vi "test-linear-system-id.vi"(8 "error in (no error)":errorcluster) -> (0 "error out":errorcluster, 3 "All tests passed":bool)   [LabVIEW 2019]
uses:
  <vilib>/Rock Robotics/WPI/ThirdParty/JAS_Junk/TrajLib/LINEAR_SYSTEM.ctl
  <vilib>/Analysis/Matrix/Datatypes/RealMatrix.ctl
  <vilib>/Rock Robotics/WPI/ThirdParty/JAS_Junk/TrajLib/MatBuilder_Create.vi
  <vilib>/Rock Robotics/WPI/ThirdParty/JAS_Junk/TrajLib/LinearSystem_New.vi
  <vilib>/Rock Robotics/WPI/ThirdParty/JAS_Junk/TrajLib/MatrixHelper_Zero.vi
  <vilib>/Rock Robotics/WPI/ThirdParty/JAS_Junk/TrajLib/DCMotor_New.vi
  <vilib>/Rock Robotics/WPI/ThirdParty/JAS_Junk/TrajLib/Units_RotationsPerMinuteToRadiansPerSecond.vi
  <vilib>/Rock Robotics/WPI/ThirdParty/JAS_Junk/TrajLib/MatrixHelper_CoerceSize.vi
  <vilib>/Analysis/7linalg.llb/Create Special Matrix.vi
  <vilib>/Analysis/7linalg.llb/Create Special Real Matrix.vi
  <vilib>/Rock Robotics/WPI/ThirdParty/JAS_Junk/TrajLib/Trajectory_Library.lvlib
  <vilib>/Analysis/Matrix/NI_Matrix.lvlib
panel:
  out "T D 6":bool
  out "T C 6":bool
  out "T B 6":bool
  out "T A 6":bool
  out "DCMotorSystem":T1
  out "T B 5":bool
  out "T A 5":bool
  out "T B 4":bool
  out "T A 4":bool
  out "T D 3":bool
  out "T C 3":bool
  out "T B 3":bool
  out "T A 3":bool
  out "T D 2":bool
  out "T C 2":bool
  out "T B 2":bool
  out "T A 2":bool
  out "T D 1":bool
  out "T C 1":bool
  out "T B 1":bool
  out "T A 1":bool
  out "IdentifyVelocitySystem":T1
  out "IdentifyPositionSystem":T1
  out "FlyWheel":T1
  out "DriveTrain":T1
  out "Elevator":T1
  # "A  = -10.14132, 3.06598, \n            3.06598, -10.14132\n\nB =    4.2590,   -1.28762, \n         -1.2876,   4.2590\n\nC =   1.0,   0.0, \n          0.0,  1.0;\n\nD =   0.0,   0.0, \n          0.0,   0.0"
  # "A   = (0, 1, \n               0, -99.05473)\n\n     B = (0, \n            20.8)\n\n   C   = 1, 0\n\n    D = 0"
  # "A = -26.87032\n\nB = 1354.166667;\n\nC = 1\n\nD = 0"
  # "A =   0, 1, \n         0, -1 / 0.5\n\nB =  0, \n        1 / 0.5"
  # "A =   -1.0 / 0.5\n\nB = 1 / 0.5"
  # "<States,States>"
  # "<States,Inputs>"
  # "<Outputs,States>"
  # "<Outputs,Inputs>"
  # "<States,States>"
  # "<States,Inputs>"
  # "<Outputs,States>"
  # "<Outputs,Inputs>"
  # "<States,States>"
  # "<States,Inputs>"
  # "<Outputs,States>"
  # "<Outputs,Inputs>"
  # "<States,States>"
  # "<States,Inputs>"
  # "<Outputs,States>"
  # "<Outputs,Inputs>"
  # "<States,States>"
  # "<States,Inputs>"
  # "<Outputs,States>"
  # "<Outputs,Inputs>"
  # "<States,States>"
  # "<States,Inputs>"
  # "<Outputs,States>"
  # "<Outputs,Inputs>"
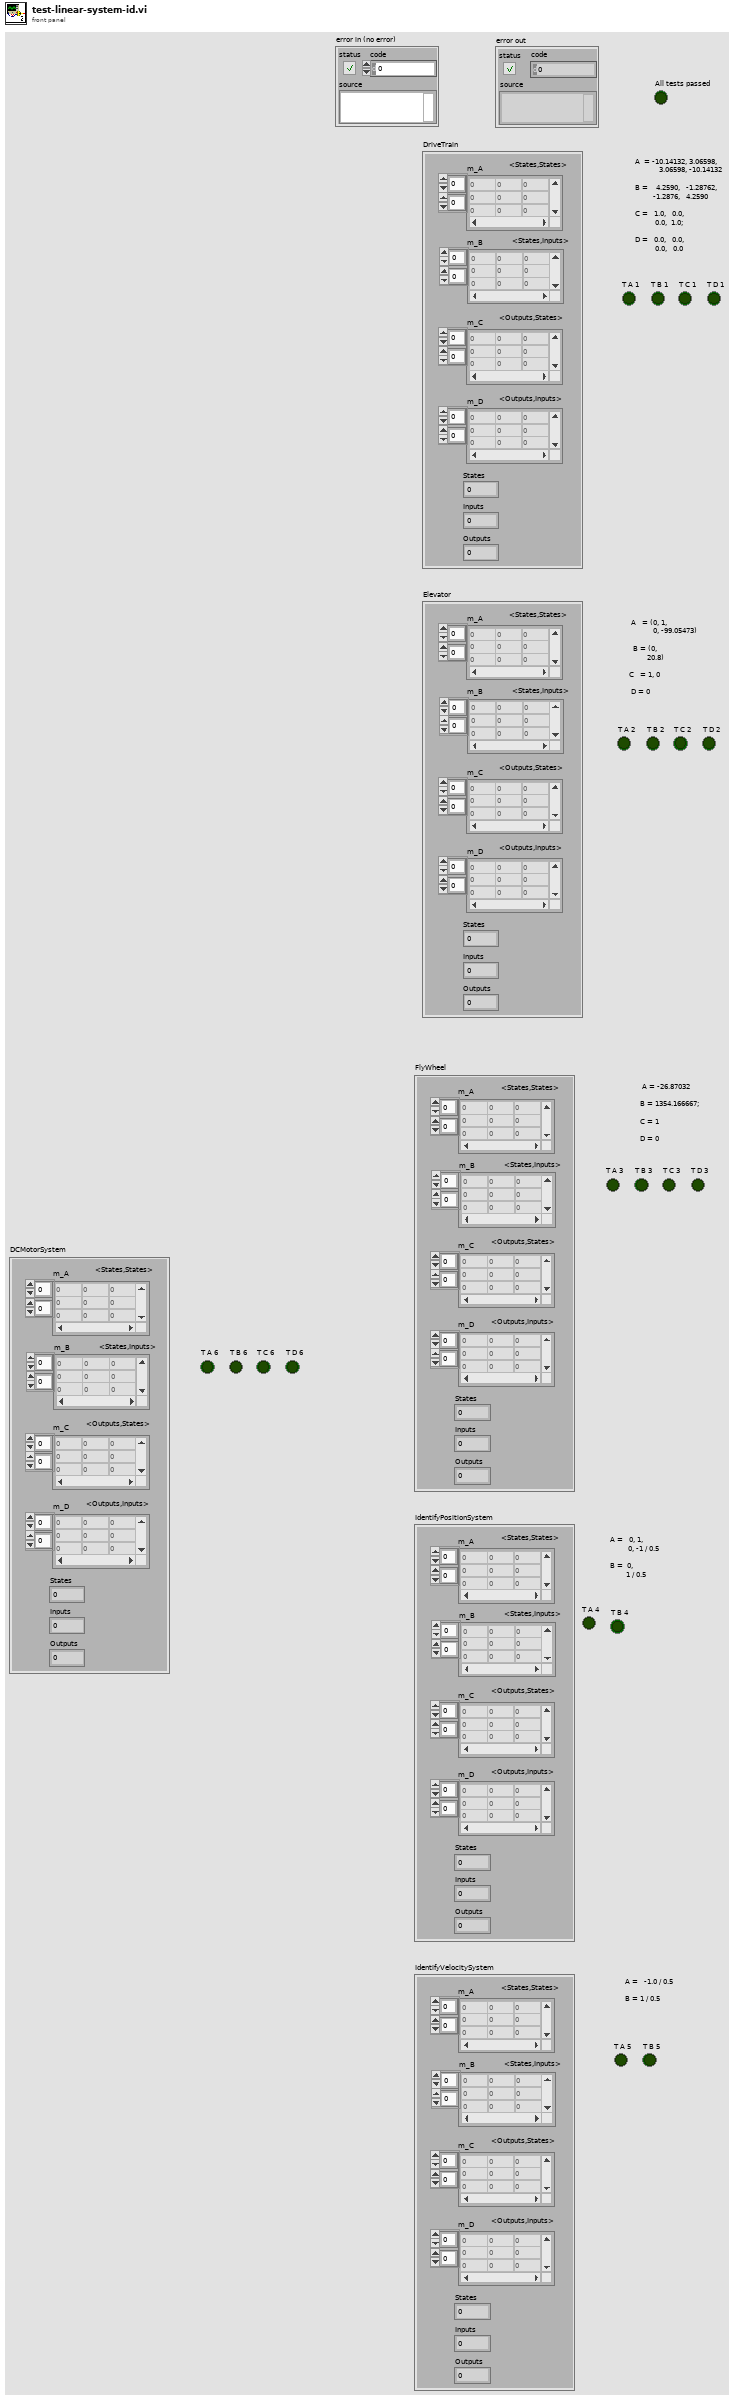
[diagram p1: front panel]
types:
  T1 = typedef "Trajectory_Library.lvlib/LINEAR_SYSTEM.ctl" = cluster{"m_A":T2, "m_B":T2, "m_C":T2, "m_D":T2, "States":i32, "Inputs":i32, "Outputs":i32}
  T2 = typedef "NI_Matrix.lvlib/RealMatrix.ctl" = dbl[][]
  T3 = typedef "Trajectory_Library.lvlib/DCMOTOR.CTL" = cluster{"nominalVoltage_Volts":dbl, "StallTorque_NM":dbl, "StallCurrent_Amps":dbl, "FreeCurrent_Amps":dbl, "FreeSpeed_RadPerSec":dbl, "R_Ohms":dbl, "KvINV_RadPerSecPerVolt":dbl, "Kt_NMPerAmp":dbl, "L_H":dbl, "Jr_KgM2":dbl}
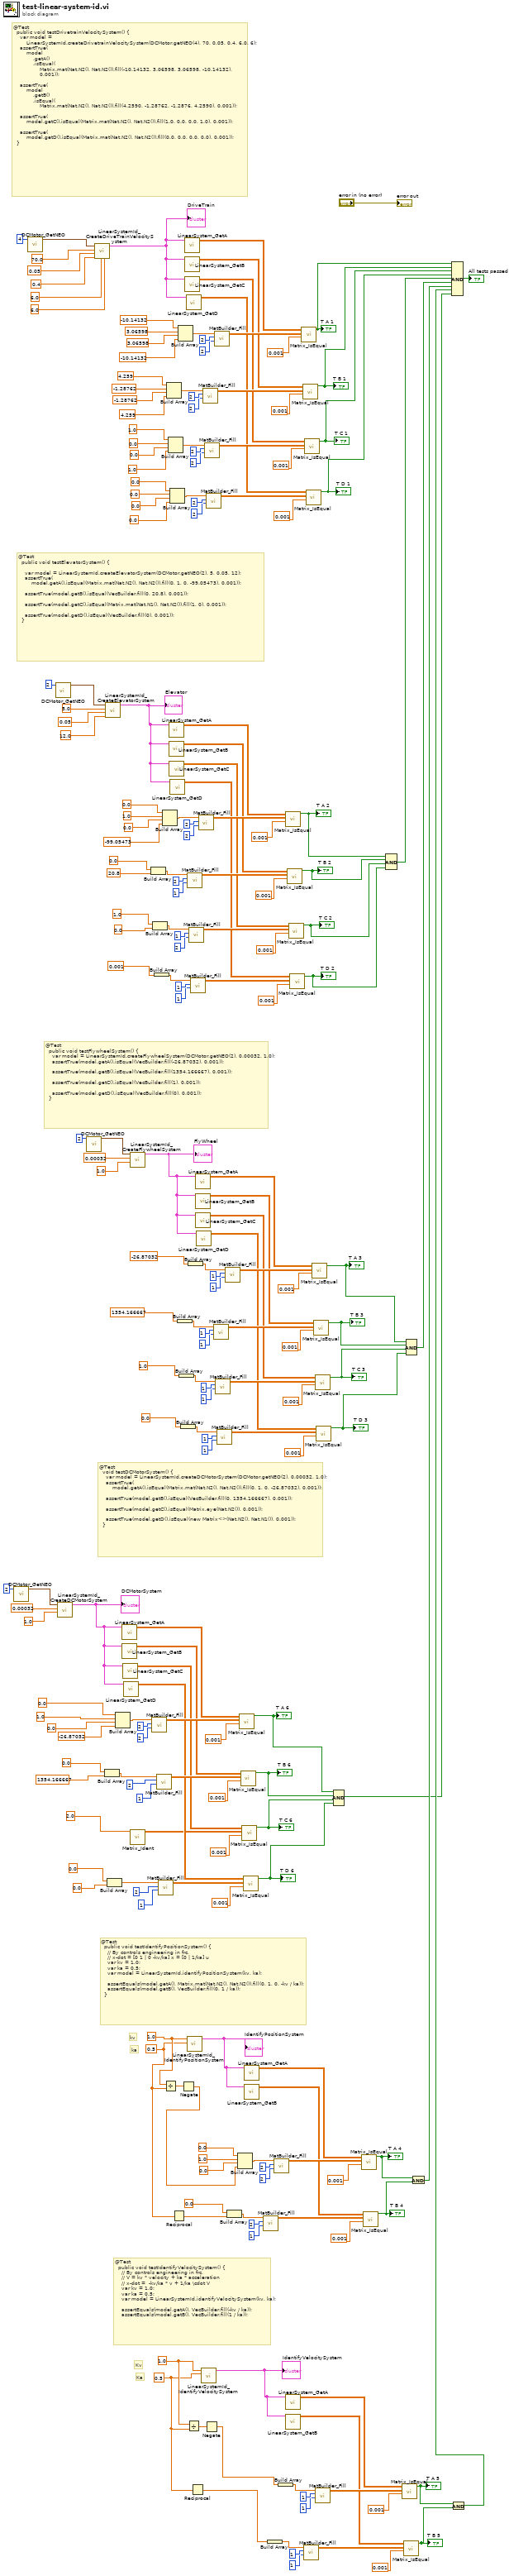
[diagram p0: block diagram]
diagram:
  w65 = 0.5 ("kA")
  w67 = 1.0 ("kV")
  w69 = 0.5 ("kA")
  w72 = 1.0 ("kV")
  # "@Test\n  void testDCMotorSystem() {\n    var model = LinearSystemId.createDCMotorSystem(DCMotor.getNEO(2), 0.00032, 1.0);\n    assertTrue(\n        model.getA().isEqual(Matrix.mat(Nat.N2(), Nat.N2()).fill(0, 1, 0, -26.87032), 0.001));\n\n    assertTrue(model.getB().isEqual(VecBuilder.fill(0, 1354.166667), 0.001));\n\n    assertTrue(model.getC().isEqual(Matrix.eye(Nat.N2()), 0.001));\n\n    assertTrue(model.getD().isEqual(new Matrix<>(Nat.N2(), Nat.N1()), 0.001));\n  }"
  # "Ka"
  # "Kv"
  # "ka"
  # "kv"
  # "@Test\n  public void testIdentifyVelocitySystem() {\n    // By controls engineering in frc,\n    // V = kv * velocity + ka * acceleration\n    // x-dot =  -kv/ka * v + 1/ka \\cdot V\n    var kv = 1.0;\n    var ka = 0.5;\n    var model = LinearSystemId.identifyVelocitySystem(kv, ka);\n\n    assertEquals(model.getA(), VecBuilder.fill(-kv / ka));\n    assertEquals(model.getB(), VecBuilder.fill(1 / ka));"
  # "@Test\n  public void testIdentifyPositionSystem() {\n    // By controls engineering in frc,\n    // x-dot = [0 1 | 0 -kv/ka] x = [0 | 1/ka] u\n    var kv = 1.0;\n    var ka = 0.5;\n    var model = LinearSystemId.identifyPositionSystem(kv, ka);\n\n    assertEquals(model.getA(), Matrix.mat(Nat.N2(), Nat.N2()).fill(0, 1, 0, -kv / ka));\n    assertEquals(model.getB(), VecBuilder.fill(0, 1 / ka));\n  }"
  # "@Test\n  public void testFlywheelSystem() {\n    var model = LinearSystemId.createFlywheelSystem(DCMotor.getNEO(2), 0.00032, 1.0);\n    assertTrue(model.getA().isEqual(VecBuilder.fill(-26.87032), 0.001));\n\n    assertTrue(model.getB().isEqual(VecBuilder.fill(1354.166667), 0.001));\n\n    assertTrue(model.getC().isEqual(VecBuilder.fill(1), 0.001));\n\n    assertTrue(model.getD().isEqual(VecBuilder.fill(0), 0.001));\n  }"
  # "@Test\n  public void testDrivetrainVelocitySystem() {\n    var model =\n        LinearSystemId.createDrivetrainVelocitySystem(DCMotor.getNEO(4), 70, 0.05, 0.4, 6.0, 6);\n    assertTrue(\n        model\n            .getA()\n            .isEqual(\n                Matrix.mat(Nat.N2(), Nat.N2()).fill(-10.14132, 3.06598, 3.06598, -10.14132),\n                0.001));\n\n    assertTrue(\n        model\n            .getB()\n            .isEqual(\n                Matrix.mat(Nat.N2(), Nat.N2()).fill(4.2590, -1.28762, -1.2876, 4.2590), 0.001));\n\n    assertTrue(\n        model.getC().isEqual(Matrix.mat(Nat.N2(), Nat.N2()).fill(1.0, 0.0, 0.0, 1.0), 0.001));\n\n    assertTrue(\n        model.getD().isEqual(Matrix.mat(Nat.N2(), Nat.N2()).fill(0.0, 0.0, 0.0, 0.0), 0.001));\n  }"
  # "@Test\n  public void testElevatorSystem() {\n\n    var model = LinearSystemId.createElevatorSystem(DCMotor.getNEO(2), 5, 0.05, 12);\n    assertTrue(\n        model.getA().isEqual(Matrix.mat(Nat.N2(), Nat.N2()).fill(0, 1, 0, -99.05473), 0.001));\n\n    assertTrue(model.getB().isEqual(VecBuilder.fill(0, 20.8), 0.001));\n\n    assertTrue(model.getC().isEqual(Matrix.mat(Nat.N1(), Nat.N2()).fill(1, 0), 0.001));\n\n    assertTrue(model.getD().isEqual(VecBuilder.fill(0), 0.001));\n  }"
  n1 = call <vilib>:"DCMotor_GetNEO.vi"("Num Motors"=2) -> ("DCMOTOR"=w39:T3)  [unwired: 10 in]
  n2 = call <vilib>:"DCMotor_GetNEO.vi"("Num Motors"=4) -> ("DCMOTOR"=w216:T3)  [unwired: 10 in]
  n3 = call <vilib>:"DCMotor_GetNEO.vi"("Num Motors"=2) -> ("DCMOTOR"=w221:T3)  [unwired: 10 in]
  n4 = call <vilib>:"LinearSystemId_CreateDCMotorSystem.vi"("G"=1.0, "jKgMetersSquared"=0.00032, "DCMOTOR"=w39) -> ("Linearsystem"=w13:T1)  [unwired: 7 in, 1 out]
  "DCMotorSystem" <- w13
  n5 = call <vilib>:"DCMotor_GetNEO.vi"("Num Motors"=2) -> ("DCMOTOR"=w209:T3)  [unwired: 10 in]
  n6 = call <vilib>:"LinearSystemId_CreateDriveTrainVelocitySystem.vi"("G"=6.0, "JKgMetersSquared"=6.0, "rbMeters"=0.4, "rMeters"=0.05, "MassKg"=70.0, "Motor"=w216) -> ("Linearsystem"=w186:T1)  [unwired: 4 in, 1 out]
  "DriveTrain" <- w186
  n7 = Build Array(0.0 ("element"), 1354.166667 ("element")) -> (w29:dbl[])
  n8 = call <vilib>:"LinearSystemId_CreateElevatorSystem.vi"("G"=12.0, "radiusMeters"=0.05, "massKg"=5.0, "DCMOTOR"=w221) -> ("Linearsystem"=w133:T1)  [unwired: 6 in, 1 out]
  "Elevator" <- w133
  n9 = Build Array(0.0 ("element"), 0.0 ("element")) -> (w21:dbl[])
  n10 = Build Array(0.0 ("element"), 1.0 ("element"), 0.0 ("element"), -26.87032 ("element")) -> (w36:dbl[])
  n11 = call <vilib>:"LinearSystem_GetA.vi"("Linearsystem"=w13) -> ("A"=w32:T2)  [unwired: 10 in]
  n12 = call <vilib>:"LinearSystem_GetB.vi"("Linearsystem"=w13) -> ("B"=w23:T2)  [unwired: 10 in]
  n13 = call <vilib>:"LinearSystem_GetC.vi"("Linearsystem"=w13) -> ("C"=w15:T2)  [unwired: 10 in]
  n14 = call <vilib>:"LinearSystem_GetD.vi"("Linearsystem"=w13) -> ("D"=w14:T2)  [unwired: 10 in]
  n15 = call <vilib>:"LinearSystemId_CreateFlywheelSystem.vi"("G"=1.0, "jKgMetersSquared"=0.00032, "DCMOTOR"=w209) -> ("Linearsystem"=w104:T1)  [unwired: 7 in, 1 out]
  "FlyWheel" <- w104
  n16 = call <vilib>:"Matrix_Ident.vi"("Size"=2.0 ("element")) -> ("output matrix"=w4:T2)  [unwired: 9 in, 1 out]
  n17 = Build Array(0.0 ("element"), 20.8 ("element")) -> (w155:dbl[])
  n18 = call <vilib>:"MatBuilder_Fill.vi"("Columns"=2, "Rows"=2, "Value List"=w36) -> ("output matrix"=w31:T2)  [unwired: 8 in]
  n19 = Build Array(1.0 ("element"), 0.0 ("element")) -> (w147:dbl[])
  n20 = Build Array(0.001 ("element")) -> (w141:dbl[])
  n21 = call <vilib>:"MatBuilder_Fill.vi"("Columns"=1, "Rows"=2, "Value List"=w29) -> ("output matrix"=w25:T2)  [unwired: 8 in]
  n22 = call <vilib>:"MatBuilder_Fill.vi"("Columns"=1, "Rows"=2, "Value List"=w21) -> ("output matrix"=w17:T2)  [unwired: 8 in]
  n23 = Build Array(0.0 ("element"), 1.0 ("element"), 0.0 ("element"), -99.05473 ("element")) -> (w165:dbl[])
  n24 = Divide(x=w72, y=w69) -> (x/y=w73:dbl)
  n25 = Build Array(4.259 ("element"), -1.28762 ("element"), -1.28762 ("element"), 4.259 ("element")) -> (w196:dbl[])
  n26 = Build Array(1.0 ("element"), 0.0 ("element"), 0.0 ("element"), 1.0 ("element")) -> (w185:dbl[])
  n27 = call <vilib>:"LinearSystem_GetA.vi"("Linearsystem"=w133) -> ("A"=w158:T2)  [unwired: 10 in]
  n28 = call <vilib>:"LinearSystem_GetB.vi"("Linearsystem"=w133) -> ("B"=w148:T2)  [unwired: 10 in]
  n29 = call <vilib>:"LinearSystem_GetC.vi"("Linearsystem"=w133) -> ("C"=w135:T2)  [unwired: 10 in]
  n30 = Build Array(0.0 ("element"), 0.0 ("element"), 0.0 ("element"), 0.0 ("element")) -> (w176:dbl[])
  n31 = call <vilib>:"LinearSystem_GetD.vi"("Linearsystem"=w133) -> ("D"=w134:T2)  [unwired: 10 in]
  n32 = Reciprocal(x=w69) -> (1/x=w70:dbl)
  n33 = Build Array(1354.166667 ("element")) -> (w125:dbl[])
  n34 = Build Array(-10.14132 ("element"), 3.06598 ("element"), 3.06598 ("element"), -10.14132 ("element")) -> (w206:dbl[])
  n35 = Build Array(1.0 ("element")) -> (w118:dbl[])
  n36 = Build Array(0.0 ("element")) -> (w112:dbl[])
  n37 = Negate(x=w73) -> (-x=w71:dbl)
  n38 = call <vilib>:"LinearSystem_GetA.vi"("Linearsystem"=w186) -> ("A"=w199:T2)  [unwired: 10 in]
  n39 = call <vilib>:"LinearSystem_GetB.vi"("Linearsystem"=w186) -> ("B"=w187:T2)  [unwired: 10 in]
  n40 = call <vilib>:"LinearSystem_GetC.vi"("Linearsystem"=w186) -> ("C"=w167:T2)  [unwired: 10 in]
  n41 = call <vilib>:"LinearSystem_GetD.vi"("Linearsystem"=w186) -> ("D"=w166:T2)  [unwired: 10 in]
  n42 = Divide(x=w67, y=w65) -> (x/y=w68:dbl)
  n43 = call <vilib>:"LinearSystemId_IdentifyPositionSystem.vi"("kA"=w69, "kV"=w72) -> ("Linearsystem"=w87:T1)  [unwired: 8 in, 1 out]
  "IdentifyPositionSystem" <- w87
  n44 = call <vilib>:"MatBuilder_Fill.vi"("Columns"=1, "Rows"=2, "Value List"=w155) -> ("output matrix"=w150:T2)  [unwired: 8 in]
  n45 = Build Array(-26.87032 ("element")) -> (w132:dbl[])
  n46 = call <vilib>:"MatBuilder_Fill.vi"("Columns"=2, "Rows"=1, "Value List"=w147) -> ("output matrix"=w143:T2)  [unwired: 8 in]
  n47 = call <vilib>:"MatBuilder_Fill.vi"("Columns"=1, "Rows"=1, "Value List"=w141) -> ("output matrix"=w137:T2)  [unwired: 8 in]
  n48 = Reciprocal(x=w65) -> (1/x=w63:dbl)
  n49 = call <vilib>:"LinearSystem_GetA.vi"("Linearsystem"=w104) -> ("A"=w128:T2)  [unwired: 10 in]
  n50 = call <vilib>:"LinearSystem_GetB.vi"("Linearsystem"=w104) -> ("B"=w119:T2)  [unwired: 10 in]
  n51 = call <vilib>:"LinearSystem_GetC.vi"("Linearsystem"=w104) -> ("C"=w106:T2)  [unwired: 10 in]
  n52 = call <vilib>:"LinearSystem_GetD.vi"("Linearsystem"=w104) -> ("D"=w105:T2)  [unwired: 10 in]
  n53 = call <vilib>:"MatBuilder_Fill.vi"("Columns"=2, "Rows"=2, "Value List"=w165) -> ("output matrix"=w157:T2)  [unwired: 8 in]
  n54 = call <vilib>:"LinearSystemId_IdentifyVelocitySystem.vi"("kA"=w65, "kV"=w67) -> ("Linearsystem"=w75:T1)  [unwired: 8 in, 1 out]
  "IdentifyVelocitySystem" <- w75
  n55 = call <vilib>:"MatBuilder_Fill.vi"("Columns"=2, "Rows"=2, "Value List"=w196) -> ("output matrix"=w189:T2)  [unwired: 8 in]
  n56 = Negate(x=w68) -> (-x=w66:dbl)
  n57 = call <vilib>:"MatBuilder_Fill.vi"("Columns"=2, "Rows"=2, "Value List"=w185) -> ("output matrix"=w178:T2)  [unwired: 8 in]
  n58 = call <vilib>:"MatBuilder_Fill.vi"("Columns"=2, "Rows"=2, "Value List"=w176) -> ("output matrix"=w169:T2)  [unwired: 8 in]
  n59 = call <vilib>:"MatBuilder_Fill.vi"("Columns"=1, "Rows"=1, "Value List"=w125) -> ("output matrix"=w121:T2)  [unwired: 8 in]
  n60 = call <vilib>:"MatBuilder_Fill.vi"("Columns"=2, "Rows"=2, "Value List"=w206) -> ("output matrix"=w198:T2)  [unwired: 8 in]
  n61 = call <vilib>:"MatBuilder_Fill.vi"("Columns"=1, "Rows"=1, "Value List"=w118) -> ("output matrix"=w114:T2)  [unwired: 8 in]
  n62 = call <vilib>:"MatBuilder_Fill.vi"("Columns"=1, "Rows"=1, "Value List"=w112) -> ("output matrix"=w108:T2)  [unwired: 8 in]
  n63 = call <vilib>:"MatBuilder_Fill.vi"("Columns"=1, "Rows"=1, "Value List"=w132) -> ("output matrix"=w127:T2)  [unwired: 8 in]
  n64 = Build Array(0.0 ("element"), w70) -> (w94:dbl[])
  n65 = Build Array(0.0 ("element"), 1.0 ("element"), 0.0 ("element"), w71) -> (w103:dbl[])
  n66 = call <vilib>:"Matrix_IsEqual.vi"("Tolerance"=0.001, "other"=w31, "input matrix"=w32) -> ("Equal"=w12:bool)  [unwired: 8 in]
  "T A 6" <- w12
  n67 = call <vilib>:"Matrix_IsEqual.vi"("Tolerance"=0.001, "other"=w25, "input matrix"=w23) -> ("Equal"=w11:bool)  [unwired: 8 in]
  "T B 6" <- w11
  n68 = call <vilib>:"Matrix_IsEqual.vi"("Tolerance"=0.001, "other"=w4, "input matrix"=w15) -> ("Equal"=w10:bool)  [unwired: 8 in]
  "T C 6" <- w10
  n69 = call <vilib>:"Matrix_IsEqual.vi"("Tolerance"=0.001, "other"=w17, "input matrix"=w14) -> ("Equal"=w9:bool)  [unwired: 8 in]
  "T D 6" <- w9
  n70 = call <vilib>:"LinearSystem_GetA.vi"("Linearsystem"=w87) -> ("A"=w97:T2)  [unwired: 10 in]
  n71 = call <vilib>:"LinearSystem_GetB.vi"("Linearsystem"=w87) -> ("B"=w88:T2)  [unwired: 10 in]
  n72 = call <vilib>:"MatBuilder_Fill.vi"("Columns"=1, "Rows"=2, "Value List"=w94) -> ("output matrix"=w90:T2)  [unwired: 8 in]
  n73 = Build Array(w63) -> (w64:dbl[])
  n74 = call <vilib>:"MatBuilder_Fill.vi"("Columns"=2, "Rows"=2, "Value List"=w103) -> ("output matrix"=w96:T2)  [unwired: 8 in]
  n75 = Build Array(w66) -> (w86:dbl[])
  n76 = call <vilib>:"LinearSystem_GetA.vi"("Linearsystem"=w75) -> ("A"=w83:T2)  [unwired: 10 in]
  n77 = call <vilib>:"LinearSystem_GetB.vi"("Linearsystem"=w75) -> ("B"=w76:T2)  [unwired: 10 in]
  n78 = call <vilib>:"Matrix_IsEqual.vi"("Tolerance"=0.001, "other"=w157, "input matrix"=w158) -> ("Equal"=w57:bool)  [unwired: 8 in]
  "T A 2" <- w57
  n79 = call <vilib>:"Matrix_IsEqual.vi"("Tolerance"=0.001, "other"=w150, "input matrix"=w148) -> ("Equal"=w56:bool)  [unwired: 8 in]
  "T B 2" <- w56
  n80 = call <vilib>:"Matrix_IsEqual.vi"("Tolerance"=0.001, "other"=w143, "input matrix"=w135) -> ("Equal"=w55:bool)  [unwired: 8 in]
  "T C 2" <- w55
  n81 = call <vilib>:"Matrix_IsEqual.vi"("Tolerance"=0.001, "other"=w137, "input matrix"=w134) -> ("Equal"=w54:bool)  [unwired: 8 in]
  "T D 2" <- w54
  n82 = call <vilib>:"Matrix_IsEqual.vi"("Tolerance"=0.001, "other"=w198, "input matrix"=w199) -> ("Equal"=w61:bool)  [unwired: 8 in]
  "T A 1" <- w61
  n83 = call <vilib>:"Matrix_IsEqual.vi"("Tolerance"=0.001, "other"=w189, "input matrix"=w187) -> ("Equal"=w60:bool)  [unwired: 8 in]
  "T B 1" <- w60
  n84 = call <vilib>:"MatBuilder_Fill.vi"("Columns"=1, "Rows"=1, "Value List"=w64) -> ("output matrix"=w78:T2)  [unwired: 8 in]
  n85 = call <vilib>:"Matrix_IsEqual.vi"("Tolerance"=0.001, "other"=w178, "input matrix"=w167) -> ("Equal"=w59:bool)  [unwired: 8 in]
  "T C 1" <- w59
  n86 = call <vilib>:"Matrix_IsEqual.vi"("Tolerance"=0.001, "other"=w169, "input matrix"=w166) -> ("Equal"=w58:bool)  [unwired: 8 in]
  "T D 1" <- w58
  n87 = call <vilib>:"Matrix_IsEqual.vi"("Tolerance"=0.001, "other"=w127, "input matrix"=w128) -> ("Equal"=w52:bool)  [unwired: 8 in]
  "T A 3" <- w52
  n88 = call <vilib>:"Matrix_IsEqual.vi"("Tolerance"=0.001, "other"=w121, "input matrix"=w119) -> ("Equal"=w51:bool)  [unwired: 8 in]
  "T B 3" <- w51
  n89 = call <vilib>:"Matrix_IsEqual.vi"("Tolerance"=0.001, "other"=w114, "input matrix"=w106) -> ("Equal"=w50:bool)  [unwired: 8 in]
  "T C 3" <- w50
  n90 = call <vilib>:"MatBuilder_Fill.vi"("Columns"=1, "Rows"=1, "Value List"=w86) -> ("output matrix"=w82:T2)  [unwired: 8 in]
  n91 = call <vilib>:"Matrix_IsEqual.vi"("Tolerance"=0.001, "other"=w108, "input matrix"=w105) -> ("Equal"=w49:bool)  [unwired: 8 in]
  "T D 3" <- w49
  n92 = Compound Arithmetic op=AND(w12, w11, w10, w9) -> (w1:bool)
  n93 = call <vilib>:"Matrix_IsEqual.vi"("Tolerance"=0.001, "other"=w96, "input matrix"=w97) -> ("Equal"=w47:bool)  [unwired: 8 in]
  "T A 4" <- w47
  n94 = call <vilib>:"Matrix_IsEqual.vi"("Tolerance"=0.001, "other"=w90, "input matrix"=w88) -> ("Equal"=w46:bool)  [unwired: 8 in]
  "T B 4" <- w46
  n95 = Compound Arithmetic op=AND(w57, w56, w55, w54) -> (w53:bool)
  n96 = call <vilib>:"Matrix_IsEqual.vi"("Tolerance"=0.001, "other"=w82, "input matrix"=w83) -> ("Equal"=w44:bool)  [unwired: 8 in]
  "T A 5" <- w44
  n97 = call <vilib>:"Matrix_IsEqual.vi"("Tolerance"=0.001, "other"=w78, "input matrix"=w76) -> ("Equal"=w43:bool)  [unwired: 8 in]
  "T B 5" <- w43
  n98 = Compound Arithmetic op=AND(w52, w51, w50, w49) -> (w48:bool)
  n99 = Compound Arithmetic op=AND(w47, w46) -> (w45:bool)
  n100 = Compound Arithmetic op=AND(w44, w43) -> (w42:bool)
  n101 = Compound Arithmetic op=AND(w61, w60, w59, w58, w53, w48, w45, w42, w1) -> (→"All tests passed":bool)
  "error out" <- "error in (no error)"
